vi "comDBPatientQueries.vi"(0 "id":string, 1 "State":T1, 2 "select":enum16{"Default", "Trash", "Training"}(ring), 5 "입력":string[](array[string]), 7 "searchForm":string, 9 "crrentPage":string, 11 "error in (no error)":errorcluster caption="에러 입력(에러 없음)") -> (4 "resultList":string[][](table) caption="result2DArray", 6 "result1DArray":string[](array[string]), 8 "count":i64, 15 "error out":errorcluster caption="에러 출력")   [LabVIEW 2019]
uses:
  patients_state.ctl
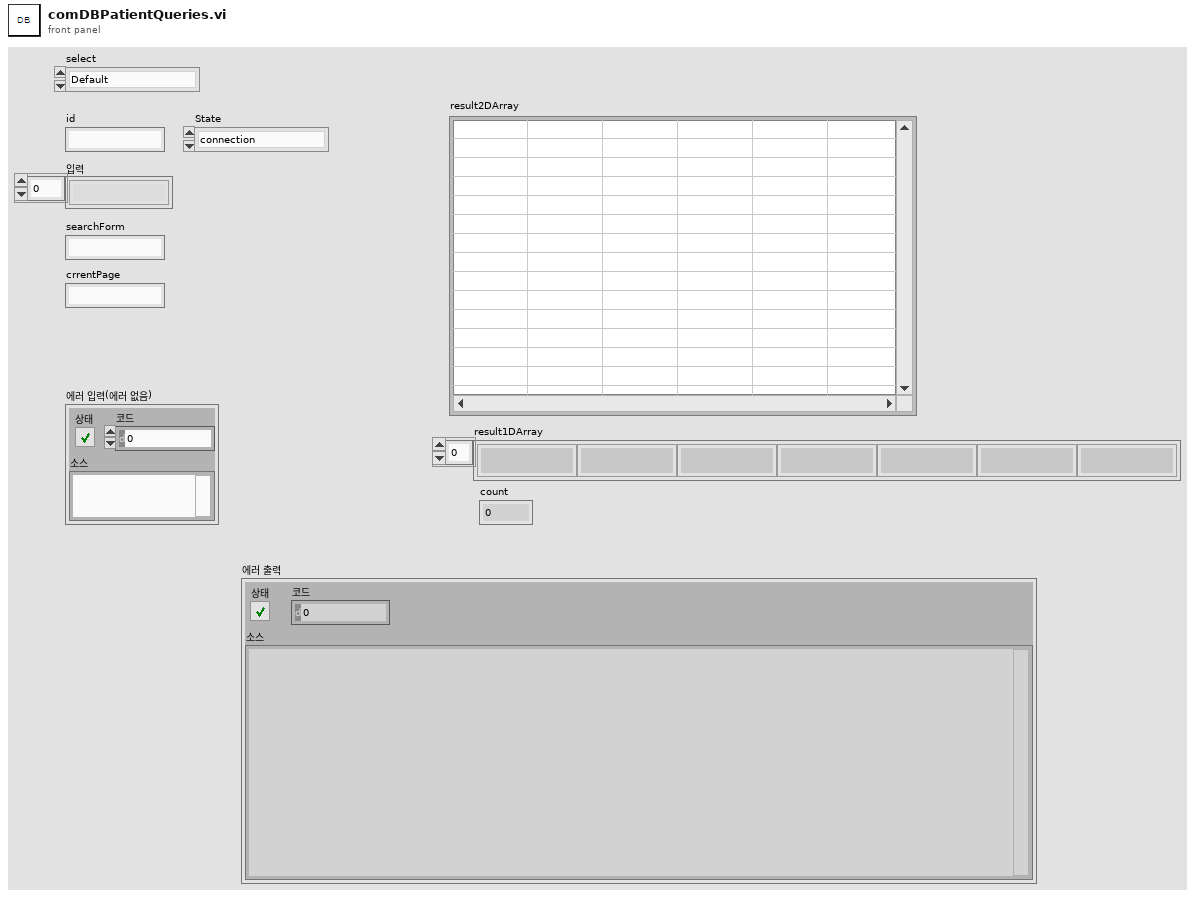
[diagram p1: front panel]
types:
  T1 = typedef "patients_state.ctl" = enum16{"connection", "create", "getReadList", "getRead", "getCount", "update", "delete", "trash", "restore", "close"}
  T2 = enum16{"connection", "create", "getReadList", "getRead", "getCount", "update", "delete", "close"}
  T3 = enum16{"connection", "create", "read", "update", "delete", "close"}
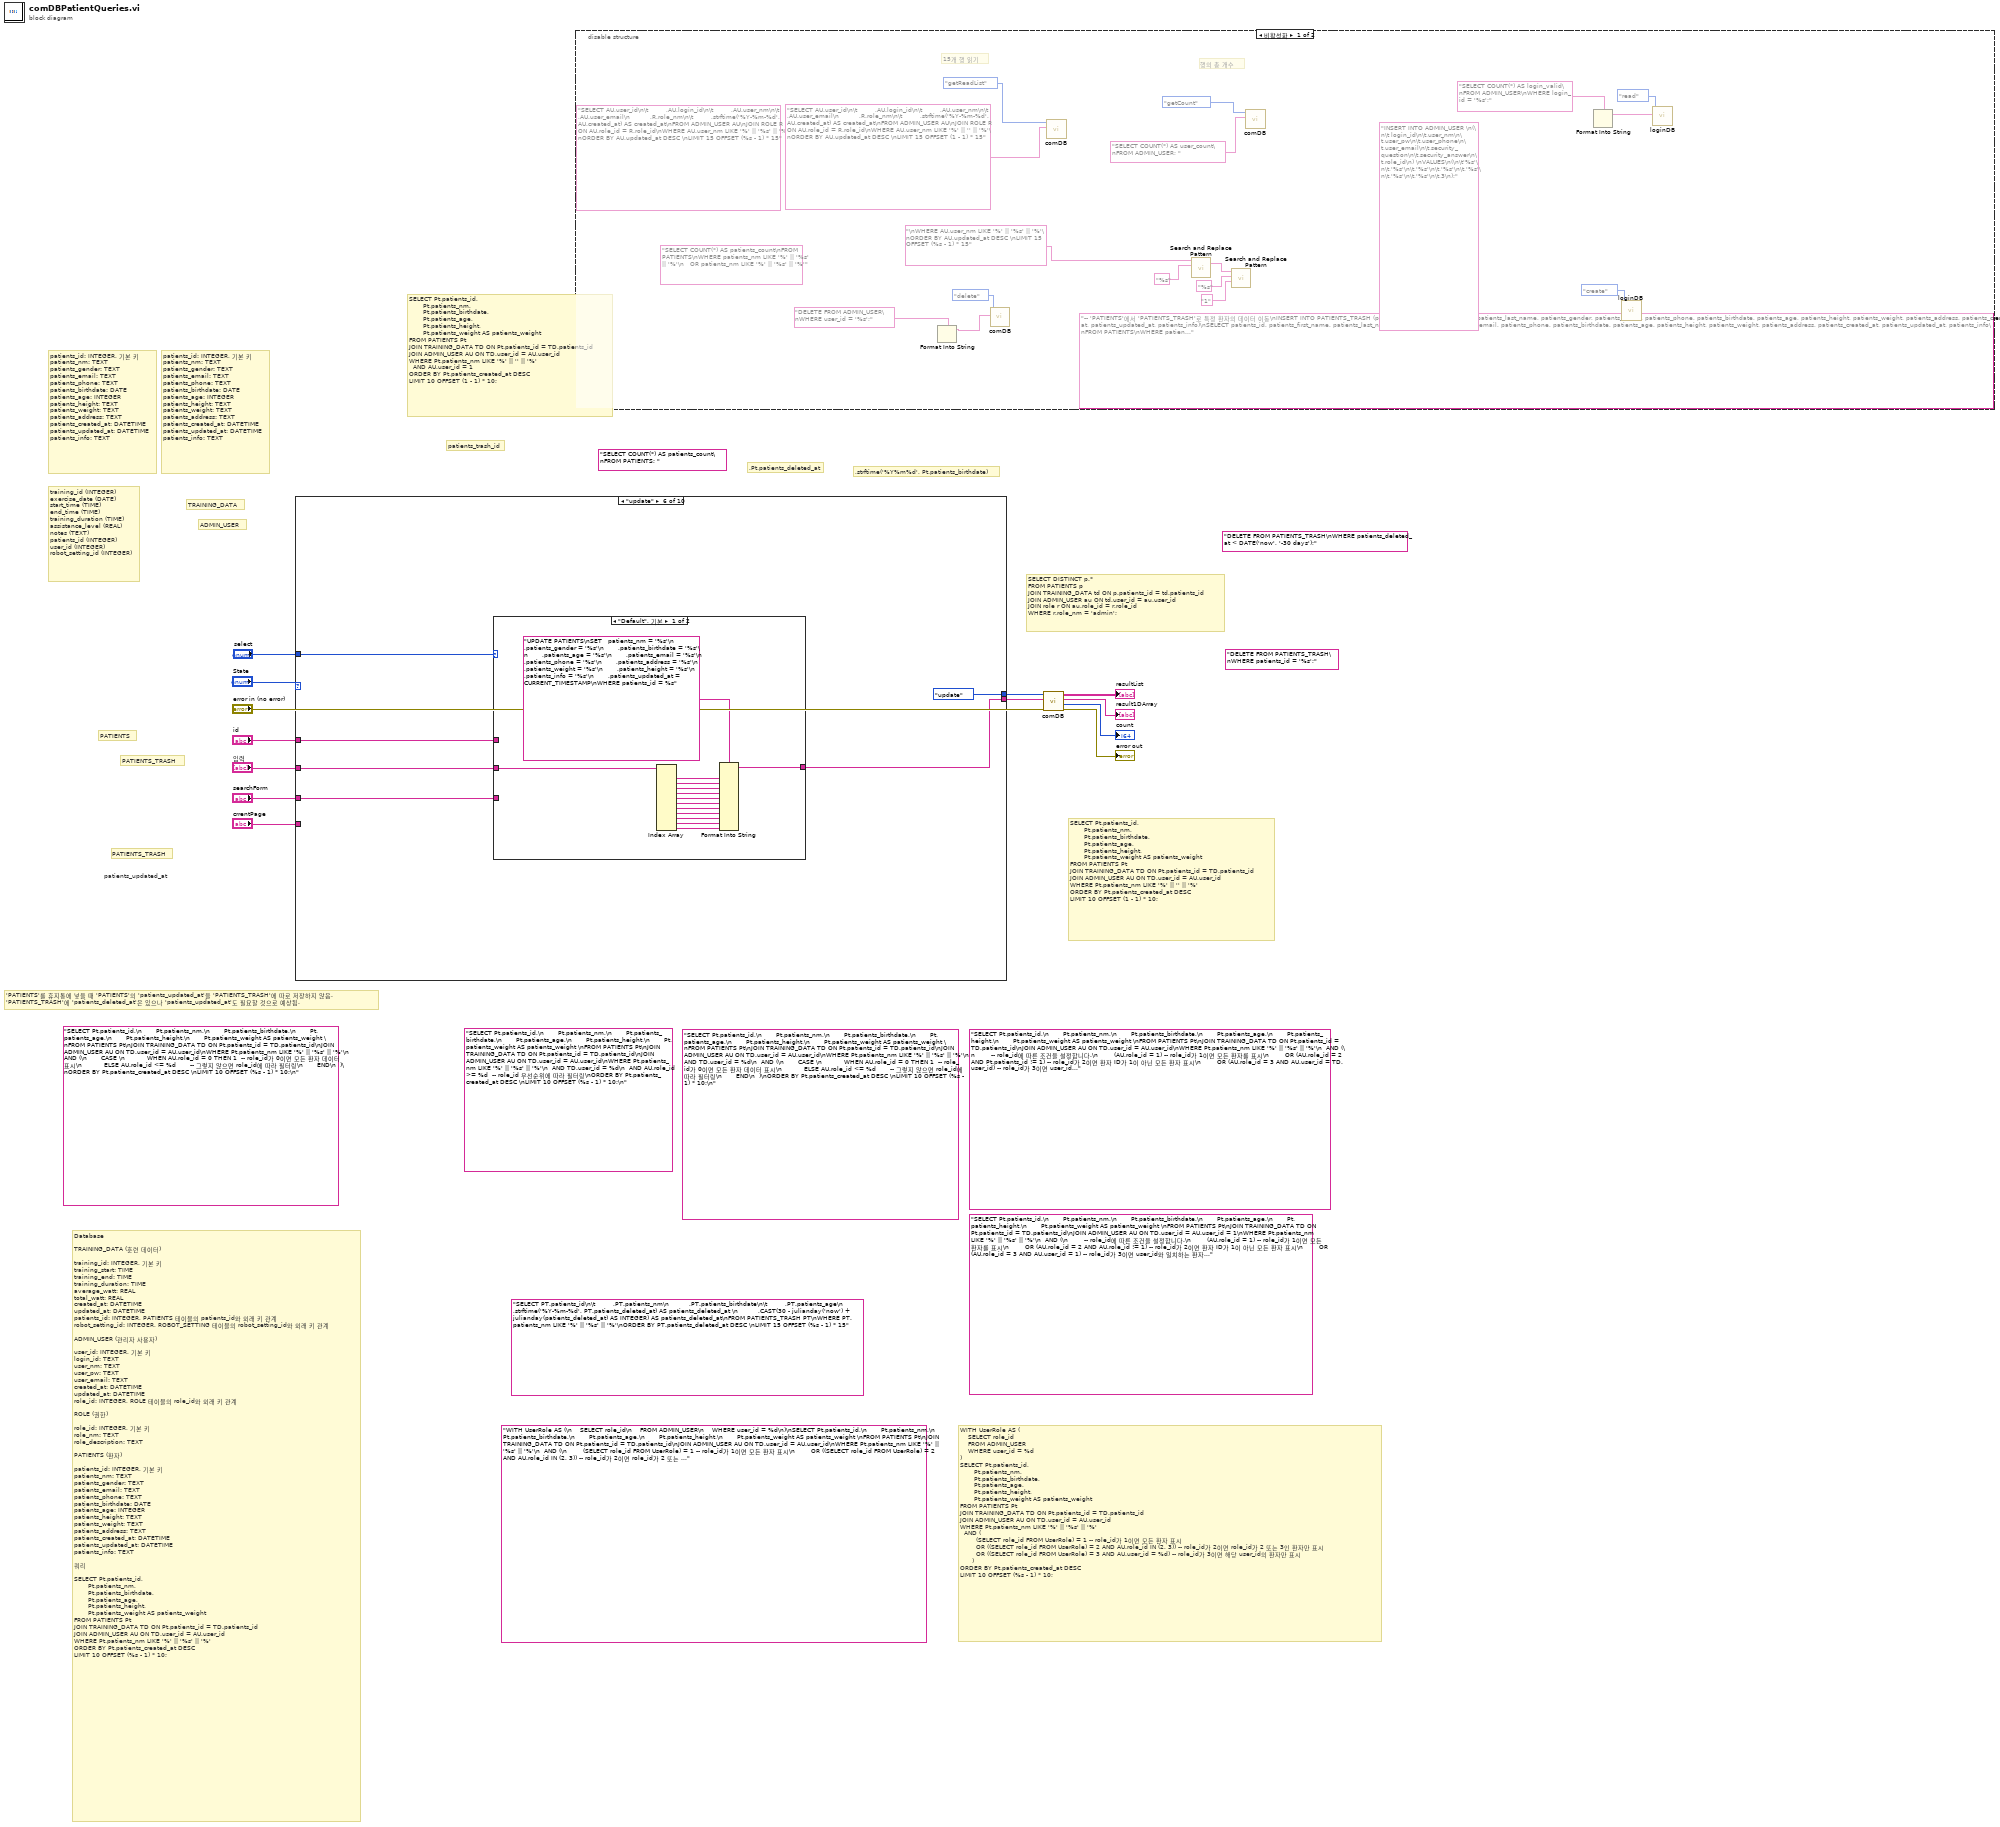
[diagram p0: block diagram]
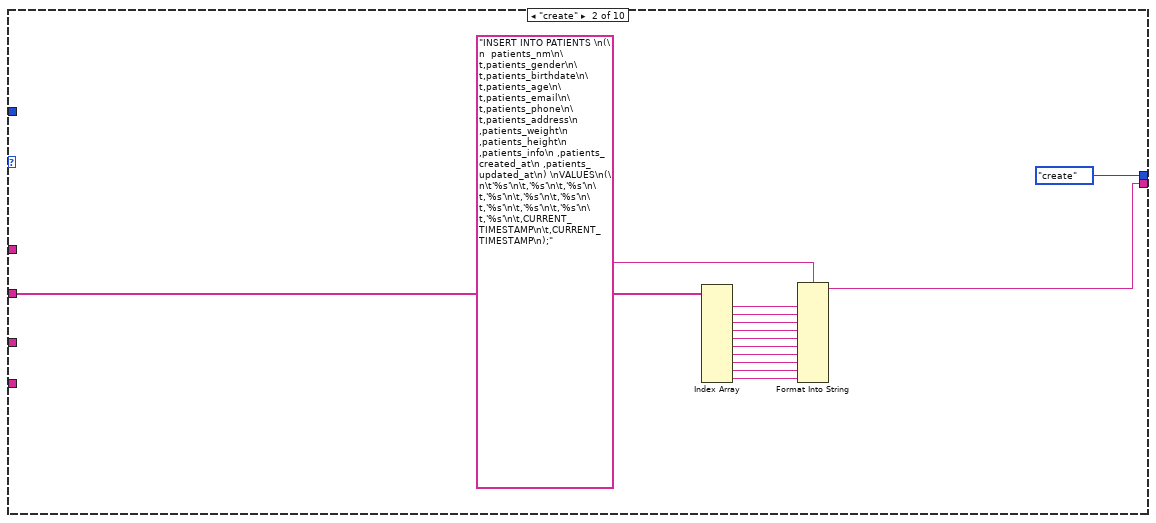
[diagram p3: hidden frame]
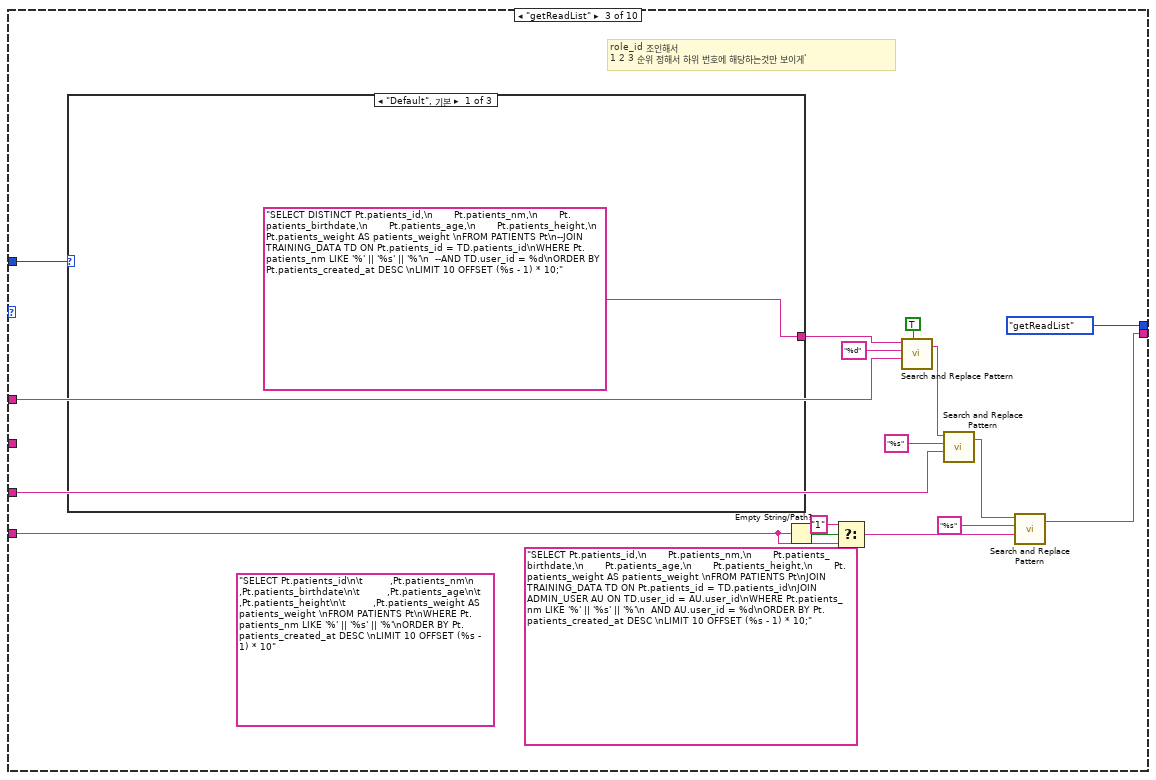
[diagram p4: hidden frame]
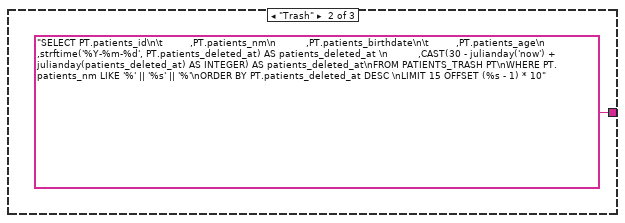
[diagram p5: hidden frame]
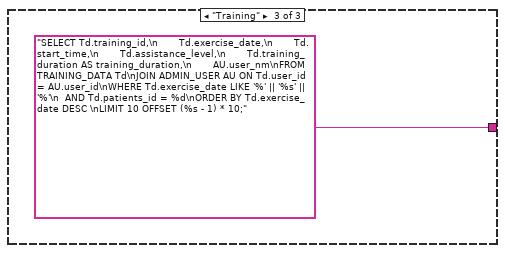
[diagram p6: hidden frame]
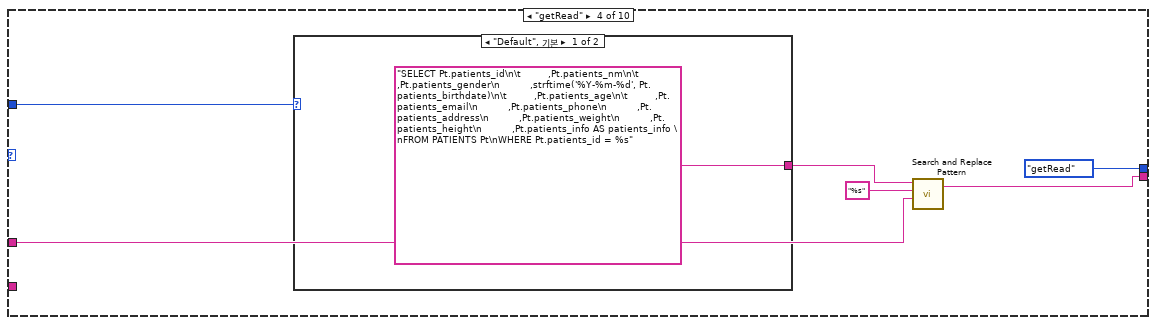
[diagram p7: hidden frame]
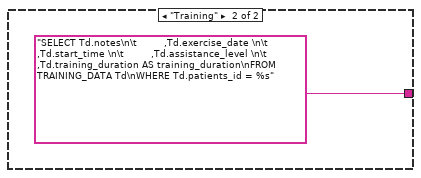
[diagram p8: hidden frame]
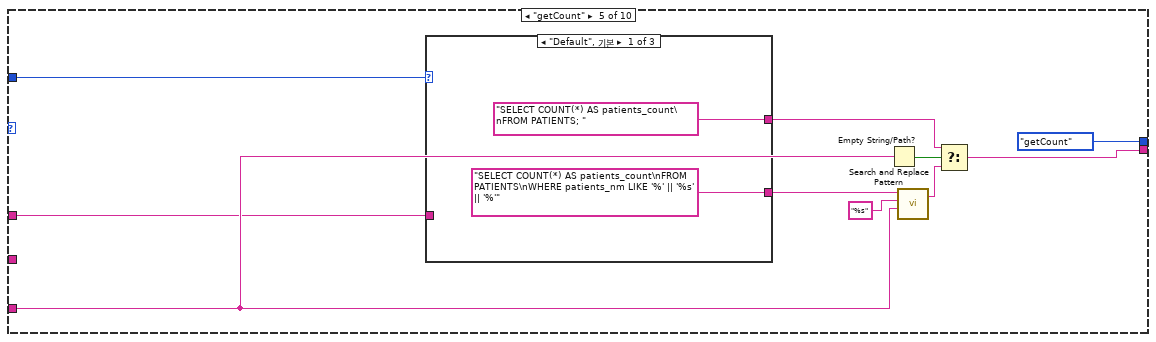
[diagram p9: hidden frame]
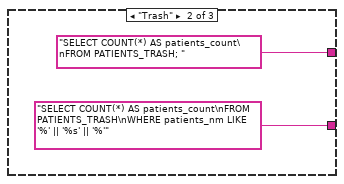
[diagram p10: hidden frame]
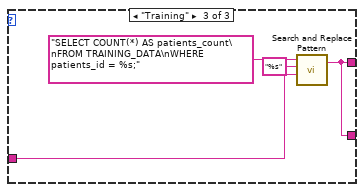
[diagram p11: hidden frame]
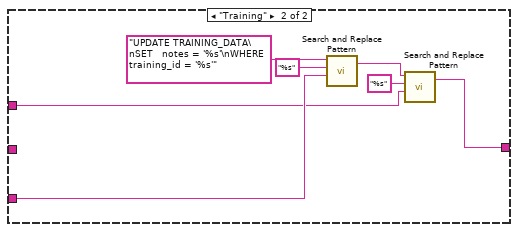
[diagram p12: hidden frame]
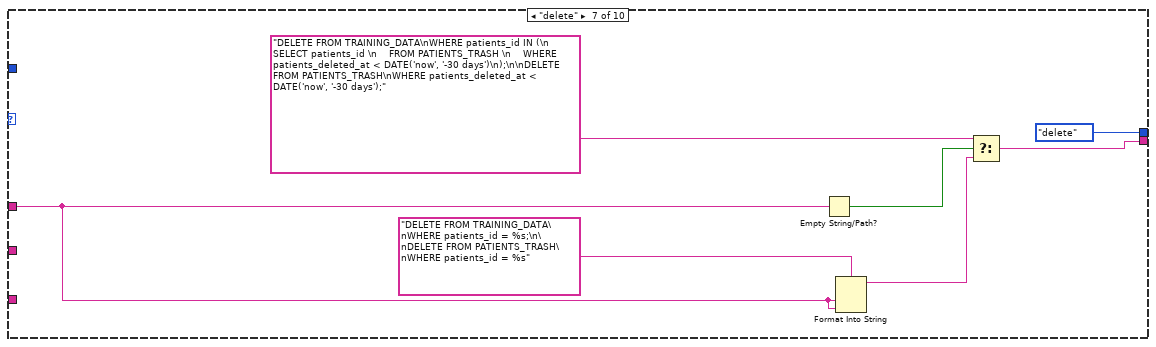
[diagram p13: hidden frame]
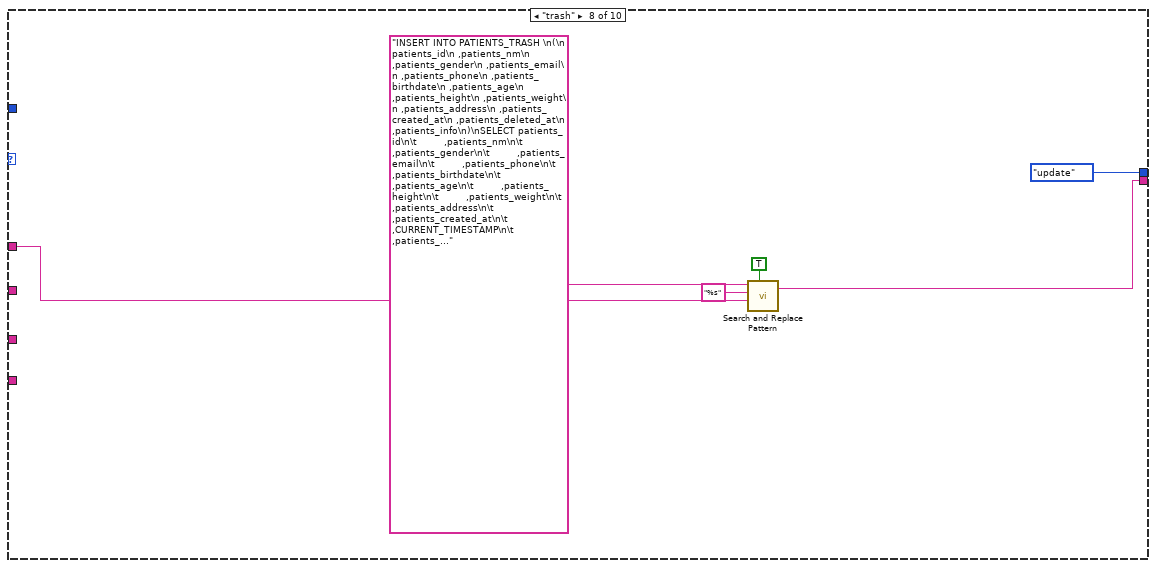
[diagram p14: hidden frame]
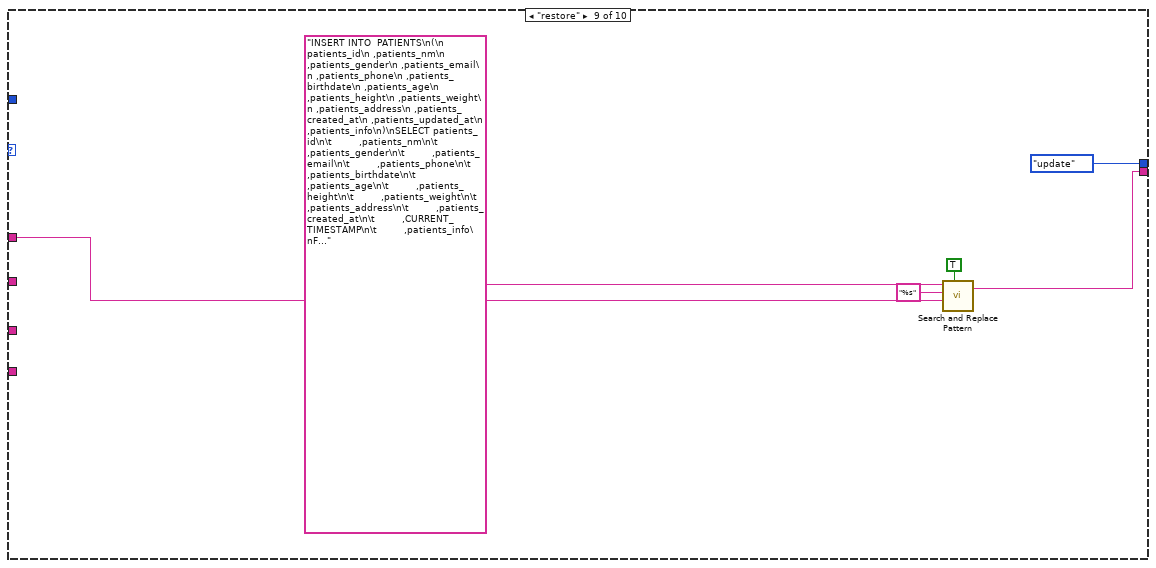
[diagram p15: hidden frame]
diagram:
  (unwired) "WITH UserRole AS (\n    SELECT role_id\n    FROM ADMIN_USER\n    WHERE user_id = %d\n)\nSELECT Pt.patients_id,\n       Pt.patients_nm,\n       Pt.patients_birthdate,\n       Pt.patients_age,\n       Pt.patients_height,\n       Pt.patients_weight AS patients_weight \nFROM PATIENTS Pt\nJOIN TRAINING_DATA TD ON Pt.patients_id = TD.patients_id\nJOIN ADMIN_USER AU ON TD.user_id = AU.user_id\nWHERE Pt.patients_nm LIKE '%' || '%s' || '%'\n  AND (\n        (SELECT role_id FROM UserRole) = 1 -- role_id가 1이면 모든 환자 표시\n        OR ((SELECT role_id FROM UserRole) = 2 AND AU.role_id IN (2, 3)) -- role_id가 2이면 role_id가 2 또는 3인 환자만 표시\n        OR ((SELECT role_id FROM UserRole) = 3 AND AU.user_id = %d) -- role_id가 3이면 해당 user_id의 환자만 표시\n      )\nORDER BY Pt.patients_created_at DESC \nLIMIT 10 OFFSET (%s - 1) * 10;\n" ("Query")
  (unwired) "SELECT PT.patients_id\n\t         ,PT.patients_nm\n          ,PT.patients_birthdate\n\t         ,PT.patients_age\n          ,strftime('%Y-%m-%d', PT.patients_deleted_at) AS patients_deleted_at \n          ,CAST(30 - julianday('now') + julianday(patients_deleted_at) AS INTEGER) AS patients_deleted_at\nFROM PATIENTS_TRASH PT\nWHERE PT.patients_nm LIKE '%' || '%s' || '%'\nORDER BY PT.patients_deleted_at DESC \nLIMIT 15 OFFSET (%s - 1) * 15" ("Query")
  (unwired) "SELECT Pt.patients_id,\n       Pt.patients_nm,\n       Pt.patients_birthdate,\n       Pt.patients_age,\n       Pt.patients_height,\n       Pt.patients_weight AS patients_weight \nFROM PATIENTS Pt\nJOIN TRAINING_DATA TD ON Pt.patients_id = TD.patients_id\nJOIN ADMIN_USER AU ON TD.user_id = AU.user_id = 1\nWHERE Pt.patients_nm LIKE '%' || '%s' || '%'\n  AND (\n        -- role_id에 따른 조건을 설정합니다.\n        (AU.role_id = 1) -- role_id가 1이면 모든 환자를 표시\n        OR (AU.role_id = 2 AND AU.role_id != 1) -- role_id가 2이면 환자 ID가 1이 아닌 모든 환자 표시\n        OR (AU.role_id = 3 AND AU.user_id = 1) -- role_id가 3이면 user_id와 일치하는 환자만 표시\n      )\nORDER BY Pt.patients_created_at DESC \nLIMIT 10 OFFSET (%s - 1) * 10;\n" ("Query")
  (unwired) "SELECT Pt.patients_id,\n       Pt.patients_nm,\n       Pt.patients_birthdate,\n       Pt.patients_age,\n       Pt.patients_height,\n       Pt.patients_weight AS patients_weight \nFROM PATIENTS Pt\nJOIN TRAINING_DATA TD ON Pt.patients_id = TD.patients_id\nJOIN ADMIN_USER AU ON TD.user_id = AU.user_id\nWHERE Pt.patients_nm LIKE '%' || '%s' || '%'\n  AND (\n        -- role_id에 따른 조건을 설정합니다.\n        (AU.role_id = 1) -- role_id가 1이면 모든 환자를 표시\n        OR (AU.role_id = 2 AND Pt.patients_id != 1) -- role_id가 2이면 환자 ID가 1이 아닌 모든 환자 표시\n        OR (AU.role_id = 3 AND AU.user_id = TD.user_id) -- role_id가 3이면 user_id와 일치하는 환자만 표시\n      )\nORDER BY Pt.patients_created_at DESC \nLIMIT 10 OFFSET (%s - 1) * 10;\n" ("Query")
  (unwired) "SELECT Pt.patients_id,\n       Pt.patients_nm,\n       Pt.patients_birthdate,\n       Pt.patients_age,\n       Pt.patients_height,\n       Pt.patients_weight AS patients_weight \nFROM PATIENTS Pt\nJOIN TRAINING_DATA TD ON Pt.patients_id = TD.patients_id\nJOIN ADMIN_USER AU ON TD.user_id = AU.user_id\nWHERE Pt.patients_nm LIKE '%' || '%s' || '%'\n  AND (\n       CASE \n           WHEN AU.role_id = 0 THEN 1  -- role_id가 0이면 모든 환자 데이터 표시\n           ELSE AU.role_id <= %d       -- 그렇지 않으면 role_id에 따라 필터링\n       END\n  )\nORDER BY Pt.patients_created_at DESC \nLIMIT 10 OFFSET (%s - 1) * 10;\n" ("Query")
  (unwired) "SELECT Pt.patients_id,\n       Pt.patients_nm,\n       Pt.patients_birthdate,\n       Pt.patients_age,\n       Pt.patients_height,\n       Pt.patients_weight AS patients_weight \nFROM PATIENTS Pt\nJOIN TRAINING_DATA TD ON Pt.patients_id = TD.patients_id\nJOIN ADMIN_USER AU ON TD.user_id = AU.user_id\nWHERE Pt.patients_nm LIKE '%' || '%s' || '%'\n  AND TD.user_id = %d\n  AND (\n       CASE \n           WHEN AU.role_id = 0 THEN 1  -- role_id가 0이면 모든 환자 데이터 표시\n           ELSE AU.role_id <= %d       -- 그렇지 않으면 role_id에 따라 필터링\n       END\n  )\nORDER BY Pt.patients_created_at DESC \nLIMIT 10 OFFSET (%s - 1) * 10;\n" ("Query")
  (unwired) "SELECT Pt.patients_id,\n       Pt.patients_nm,\n       Pt.patients_birthdate,\n       Pt.patients_age,\n       Pt.patients_height,\n       Pt.patients_weight AS patients_weight \nFROM PATIENTS Pt\nJOIN TRAINING_DATA TD ON Pt.patients_id = TD.patients_id\nJOIN ADMIN_USER AU ON TD.user_id = AU.user_id\nWHERE Pt.patients_nm LIKE '%' || '%s' || '%'\n  AND TD.user_id = %d\n  AND AU.role_id >= %d  -- role_id 우선순위에 따라 필터링\nORDER BY Pt.patients_created_at DESC \nLIMIT 10 OFFSET (%s - 1) * 10;\n" ("Query")
  (unwired) "DELETE FROM PATIENTS_TRASH\nWHERE patients_id = '%s';" ("Query")
  (unwired) "DELETE FROM PATIENTS_TRASH\nWHERE patients_deleted_at < DATE('now', '-30 days');" ("Query")
  (unwired) "SELECT COUNT(*) AS patients_count\nFROM PATIENTS; " ("Query")
  # "SELECT DISTINCT p.*\nFROM PATIENTS p\nJOIN TRAINING_DATA td ON p.patients_id = td.patients_id\nJOIN ADMIN_USER au ON td.user_id = au.user_id\nJOIN role r ON au.role_id = r.role_id\nWHERE r.role_nm = 'admin';"
  # "X"
  # "X"
  # "X"
  # "X"
  # "X"
  # "X"
  # "SELECT Pt.patients_id,\n       Pt.patients_nm,\n       Pt.patients_birthdate,\n       Pt.patients_age,\n       Pt.patients_height,\n       Pt.patients_weight AS patients_weight \nFROM PATIENTS Pt\nJOIN TRAINING_DATA TD ON Pt.patients_id = TD.patients_id\nJOIN ADMIN_USER AU ON TD.user_id = AU.user_id\nWHERE Pt.patients_nm LIKE '%' || '' || '%'\nORDER BY Pt.patients_created_at DESC \nLIMIT 10 OFFSET (1 - 1) * 10;"
  # "WITH UserRole AS (\n    SELECT role_id\n    FROM ADMIN_USER\n    WHERE user_id = %d\n)\nSELECT Pt.patients_id,\n       Pt.patients_nm,\n       Pt.patients_birthdate,\n       Pt.patients_age,\n       Pt.patients_height,\n       Pt.patients_weight AS patients_weight \nFROM PATIENTS Pt\nJOIN TRAINING_DATA TD ON Pt.patients_id = TD.patients_id\nJOIN ADMIN_USER AU ON TD.user_id = AU.user_id\nWHERE Pt.patients_nm LIKE '%' || '%s' || '%'\n  AND (\n        (SELECT role_id FROM UserRole) = 1 -- role_id가 1이면 모든 환자 표시\n        OR ((SELECT role_id FROM UserRole) = 2 AND AU.role_id IN (2, 3)) -- role_id가 2이면 role_id가 2 또는 3인 환자만 표시\n        OR ((SELECT role_id FROM UserRole) = 3 AND AU.user_id = %d) -- role_id가 3이면 해당 user_id의 환자만 표시\n      )\nORDER BY Pt.patients_created_at DESC \nLIMIT 10 OFFSET (%s - 1) * 10;"
  # "Database\n\nTRAINING_DATA (훈련 데이터)\n\ntraining_id: INTEGER, 기본 키\ntraining_start: TIME\ntraining_end: TIME\ntraining_duration: TIME\naverage_watt: REAL\ntotal_watt: REAL\ncreated_at: DATETIME\nupdated_at: DATETIME\npatients_id: INTEGER, PATIENTS 테이블의 patients_id와 외래 키 관계\nrobot_setting_id: INTEGER, ROBOT_SETTING 테이블의 robot_setting_id와 외래 키 관계\n\nADMIN_USER (관리자 사용자)\n\nuser_id: INTEGER, 기본 키\nlogin_id: TEXT\nuser_nm: TEXT\nuser_pw: TEXT\nuser_email: TEXT\ncreated_at: DATETIME\nupdated_at: DATETIME\nrole_id: INTEGER, ROLE 테이블의 role_id와 외래 키 관계\n\nROLE (권한)\n\nrole_id: INTEGER, 기본 키\nrole_nm: TEXT\nrole_description: TEXT\n\nPATIENTS (환자)\n\npatients_id: INTEGER, 기본 키\npatients_nm: TEXT\npatients_gender: TEXT\npatients_email: TEXT\npatients_phone: TEXT\npatients_birthdate: DATE\npatients_age: INTEGER\npatients_height: TEXT\npatients_weight: TEXT\npatients_address: TEXT\npatients_created_at: DATETIME\npatients_updated_at: DATETIME\npatients_info: TEXT\n\n쿼리\n\nSELECT Pt.patients_id,\n       Pt.patients_nm,\n       Pt.patients_birthdate,\n       Pt.patients_age,\n       Pt.patients_height,\n       Pt.patients_weight AS patients_weight \nFROM PATIENTS Pt\nJOIN TRAINING_DATA TD ON Pt.patients_id = TD.patients_id\nJOIN ADMIN_USER AU ON TD.user_id = AU.user_id\nWHERE Pt.patients_nm LIKE '%' || '%s' || '%'\nORDER BY Pt.patients_created_at DESC \nLIMIT 10 OFFSET (%s - 1) * 10;"
  # "SELECT Pt.patients_id,\n       Pt.patients_nm,\n       Pt.patients_birthdate,\n       Pt.patients_age,\n       Pt.patients_height,\n       Pt.patients_weight AS patients_weight \nFROM PATIENTS Pt\nJOIN TRAINING_DATA TD ON Pt.patients_id = TD.patients_id\nJOIN ADMIN_USER AU ON TD.user_id = AU.user_id\nWHERE Pt.patients_nm LIKE '%' || '' || '%'\n  AND AU.user_id = 1\nORDER BY Pt.patients_created_at DESC \nLIMIT 10 OFFSET (1 - 1) * 10;"
  # "ADMIN_USER"
  # "patients_trash_id"
  # "TRAINING_DATA"
  # "training_id (INTEGER)\nexercise_date (DATE)\nstart_time (TIME)\nend_time (TIME)\ntraining_duration (TIME)\nassistance_level (REAL)\nnotes (TEXT)\npatients_id (INTEGER)\nuser_id (INTEGER)\nrobot_setting_id (INTEGER)"
  # ",Pt.patients_deleted_at"
  # ",strftime('%Y%m%d', Pt.patients_birthdate)"
  # "patients_updated_at"
  # "PATIENTS_TRASH"
  # "'PATIENTS'를 휴지통에 넣을 때 'PATIENTS'의 'patients_updated_at'을 'PATIENTS_TRASH'에 따로 저장하지 않음.\n'PATIENTS_TRASH'에 'patients_deleted_at'은 있으나 'patients_updated_at'도 필요할 것으로 예상됨."
  # "patients_id: INTEGER, 기본 키\npatients_nm: TEXT\npatients_gender: TEXT\npatients_email: TEXT\npatients_phone: TEXT\npatients_birthdate: DATE\npatients_age: INTEGER\npatients_height: TEXT\npatients_weight: TEXT\npatients_address: TEXT\npatients_created_at: DATETIME\npatients_updated_at: DATETIME\npatients_info: TEXT"
  # "PATIENTS_TRASH"
  # "PATIENTS"
  # "patients_id: INTEGER, 기본 키\npatients_nm: TEXT\npatients_gender: TEXT\npatients_email: TEXT\npatients_phone: TEXT\npatients_birthdate: DATE\npatients_age: INTEGER\npatients_height: TEXT\npatients_weight: TEXT\npatients_address: TEXT\npatients_created_at: DATETIME\npatients_updated_at: DATETIME\npatients_info: TEXT"
  n1 = case shown="\"update\"" "State" {
    tunnel: [_ T2."create" ("State") T2."getReadList" ("State") T2."getRead" ("State") T2."getCount" ("State") T2."update" ("State") T2."delete" ("State") T2."update" ("State") T2."update" ("State") _] -> w11
    tunnel: [_ w17 w38 w49 w60 w76 w102 w109 w114 _] -> w10
    tunnel: "searchForm" -> [_ _ w41 _ w59 w73 _ _ _ _]
    tunnel: "crrentPage" -> [_ _ w35 _ _ _ _ _ _ _]
    tunnel: "id" -> [_ _ w30 w50 w55 w74 w100 w107 w115 _]
    tunnel: "입력" -> [_ w19 _ _ _ w77 _ _ _ _]
    tunnel: "select" -> [_ _ w33 w48 w58 w75 _ _ _ _]
    frame "connection", Default {
      # "x"
    }
    frame "create" {
      n2 = Index Array(array=w19) -> (element #1=w26:string, element #2=w25:string, element #3=w24:string, element #4=w23:string, element #5=w22:string, element #6=w21:string, element #7=w20:string, element #8=w16:string, element #9=w15:string, element #10=w14:string)  [unwired: 10 in]
      n3 = Format Into String(format string="INSERT INTO PATIENTS \n(\n  patients_nm\n\t,patients_gender\n\t,patients_birthdate\n\t,patients_age\n\t,patients_email\n\t,patients_phone\n\t,patients_address\n ,patients_weight\n ,patients_height\n ,patients_info\n ,patients_created_at\n ,patients_updated_at\n) \nVALUES\n(\n\t'%s'\n\t,'%s'\n\t,'%s'\n\t,'%s'\n\t,'%s'\n\t,'%s'\n\t,'%s'\n\t,'%s'\n\t,'%s'\n\t,'%s'\n\t,CURRENT_TIMESTAMP\n\t,CURRENT_TIMESTAMP\n);", w26, w25, w24, w23, w22, w21, w20, w16, w15, w14) -> (resulting string=w17:string)  [unwired: 2 in, 1 out]
    }
    frame "getReadList" {
      (unwired) "SELECT Pt.patients_id,\n       Pt.patients_nm,\n       Pt.patients_birthdate,\n       Pt.patients_age,\n       Pt.patients_height,\n       Pt.patients_weight AS patients_weight \nFROM PATIENTS Pt\nJOIN TRAINING_DATA TD ON Pt.patients_id = TD.patients_id\nJOIN ADMIN_USER AU ON TD.user_id = AU.user_id\nWHERE Pt.patients_nm LIKE '%' || '%s' || '%'\n  AND AU.user_id = %d\nORDER BY Pt.patients_created_at DESC \nLIMIT 10 OFFSET (%s - 1) * 10;" ("Query")
      (unwired) "SELECT Pt.patients_id\n\t         ,Pt.patients_nm\n          ,Pt.patients_birthdate\n\t         ,Pt.patients_age\n\t         ,Pt.patients_height\n\t         ,Pt.patients_weight AS patients_weight \nFROM PATIENTS Pt\nWHERE Pt.patients_nm LIKE '%' || '%s' || '%'\nORDER BY Pt.patients_created_at DESC \nLIMIT 10 OFFSET (%s - 1) * 10" ("Query")
      # "role_id 조인해서 \n1 2 3 순위 정해서 하위 번호에 해당하는것만 보이게'"
      n4 = case shown="\"Default\", 기본" w33 {
        tunnel: ["SELECT DISTINCT Pt.patients_id,\n       Pt.patients_nm,\n       Pt.patients_birthdate,\n       Pt.patients_age,\n       Pt.patients_height,\n       Pt.patients_weight AS patients_weight \nFROM PATIENTS Pt\n--JOIN TRAINING_DATA TD ON Pt.patients_id = TD.patients_id\nWHERE Pt.patients_nm LIKE '%' || '%s' || '%'\n  --AND TD.user_id = %d\nORDER BY Pt.patients_created_at DESC \nLIMIT 10 OFFSET (%s - 1) * 10;" ("Query") "SELECT PT.patients_id\n\t         ,PT.patients_nm\n          ,PT.patients_birthdate\n\t         ,PT.patients_age\n          ,strftime('%Y-%m-%d', PT.patients_deleted_at) AS patients_deleted_at \n          ,CAST(30 - julianday('now') + julianday(patients_deleted_at) AS INTEGER) AS patients_deleted_at\nFROM PATIENTS_TRASH PT\nWHERE PT.patients_nm LIKE '%' || '%s' || '%'\nORDER BY PT.patients_deleted_at DESC \nLIMIT 15 OFFSET (%s - 1) * 10" ("Query") "SELECT Td.training_id,\n       Td.exercise_date,\n       Td.start_time,\n       Td.assistance_level,\n       Td.training_duration AS training_duration,\n       AU.user_nm\nFROM TRAINING_DATA Td\nJOIN ADMIN_USER AU ON Td.user_id = AU.user_id\nWHERE Td.exercise_date LIKE '%' || '%s' || '%'\n  AND Td.patients_id = %d\nORDER BY Td.exercise_date DESC \nLIMIT 10 OFFSET (%s - 1) * 10;" ("Query")] -> w32
        frame "Default", Default {
        }
        frame "Trash" {
        }
        frame "Training" {
        }
      }
      n5 = Empty String/Path?(string/path=w35) -> (empty?=w37:bool)
      n6 = Select(t="1", s=w37, f=w35) -> (s? t:f=w36:string)
      n7 = call <vilib>:"Search and Replace Pattern.vi"("string"=w32, "regular expression (\"\")"="%d" ("regular expression (\"\")"), "replace string (\"\")"=w30, "replace all? (F)"=TRUE) -> ("result string"=w29:string)  [unwired: 1 in, 1 out]
      n8 = call <vilib>:"Search and Replace Pattern.vi"("string"=w29, "regular expression (\"\")"="%s" ("regular expression (\"\")"), "replace string (\"\")"=w41) -> ("result string"=w39:string)  [unwired: 2 in, 1 out]
      n9 = call <vilib>:"Search and Replace Pattern.vi"("string"=w39, "regular expression (\"\")"="%s" ("regular expression (\"\")"), "replace string (\"\")"=w36) -> ("result string"=w38:string)  [unwired: 2 in, 1 out]
    }
    frame "getRead" {
      n10 = case shown="\"Default\", 기본" w48 {
        tunnel: ["SELECT Pt.patients_id\n\t         ,Pt.patients_nm\n\t         ,Pt.patients_gender\n          ,strftime('%Y-%m-%d', Pt.patients_birthdate)\n\t         ,Pt.patients_age\n\t         ,Pt.patients_email\n          ,Pt.patients_phone\n          ,Pt.patients_address\n          ,Pt.patients_weight\n          ,Pt.patients_height\n          ,Pt.patients_info AS patients_info \nFROM PATIENTS Pt\nWHERE Pt.patients_id = %s" ("Query") "SELECT Td.notes\n\t         ,Td.exercise_date \n\t         ,Td.start_time \n\t         ,Td.assistance_level \n\t         ,Td.training_duration AS training_duration\nFROM TRAINING_DATA Td\nWHERE Td.patients_id = %s" ("Query")] -> w47
        frame "Default", Default {
        }
        frame "Training" {
        }
      }
      n11 = call <vilib>:"Search and Replace Pattern.vi"("string"=w47, "regular expression (\"\")"="%s" ("regular expression (\"\")"), "replace string (\"\")"=w50) -> ("result string"=w49:string)  [unwired: 2 in, 1 out]
    }
    frame "getCount" {
      n12 = case shown="\"Default\", 기본" w58 {
        tunnel: ["SELECT COUNT(*) AS patients_count\nFROM PATIENTS; " ("Query") "SELECT COUNT(*) AS patients_count\nFROM PATIENTS_TRASH; " ("Query") w69] -> w57
        tunnel: ["SELECT COUNT(*) AS patients_count\nFROM PATIENTS\nWHERE patients_nm LIKE '%' || '%s' || '%'" ("Query") "SELECT COUNT(*) AS patients_count\nFROM PATIENTS_TRASH\nWHERE patients_nm LIKE '%' || '%s' || '%'" ("Query") w69] -> w56
        tunnel: w55 -> [_ _ w70]
        frame "Default", Default {
        }
        frame "Trash" {
        }
        frame "Training" {
          n13 = call <vilib>:"Search and Replace Pattern.vi"("string"="SELECT COUNT(*) AS patients_count\nFROM TRAINING_DATA\nWHERE patients_id = %s;" ("Query"), "regular expression (\"\")"="%s" ("regular expression (\"\")"), "replace string (\"\")"=w70) -> ("result string"=w69:string)  [unwired: 2 in, 1 out]
        }
      }
      n14 = Empty String/Path?(string/path=w59) -> (empty?=w63:bool)
      n15 = call <vilib>:"Search and Replace Pattern.vi"("string"=w56, "regular expression (\"\")"="%s" ("regular expression (\"\")"), "replace string (\"\")"=w59) -> ("result string"=w61:string)  [unwired: 2 in, 1 out]
      n16 = Select(t=w57, s=w63, f=w61) -> (s? t:f=w60:string)
    }
    frame "update" {
      n17 = case shown="\"Default\", 기본" w75 {
        tunnel: w77 -> [w92 _]
        tunnel: [w83 w93] -> w76
        tunnel: w74 -> [_ w94]
        tunnel: w73 -> [_ w96]
        frame "Default", Default {
          n18 = Index Array(array=w92) -> (element #1=w91:string, element #2=w90:string, element #3=w89:string, element #4=w88:string, element #5=w87:string, element #6=w86:string, element #7=w85:string, element #8=w82:string, element #9=w81:string, element #10=w80:string, element #11=w79:string)  [unwired: 11 in]
          n19 = Format Into String(format string="UPDATE PATIENTS\nSET   patients_nm = '%s'\n       ,patients_gender = '%s'\n       ,patients_birthdate = '%s'\n       ,patients_age = '%s'\n       ,patients_email = '%s'\n       ,patients_phone = '%s'\n       ,patients_address = '%s'\n       ,patients_weight = '%s'\n       ,patients_height = '%s'\n       ,patients_info = '%s'\n       ,patients_updated_at = CURRENT_TIMESTAMP\nWHERE patients_id = %s" ("Query"), w91, w90, w89, w88, w87, w86, w85, w82, w81, w80, w79) -> (resulting string=w83:string)  [unwired: 2 in, 1 out]
        }
        frame "Training" {
          n20 = call <vilib>:"Search and Replace Pattern.vi"("string"="UPDATE TRAINING_DATA\nSET   notes = '%s'\nWHERE training_id = '%s'" ("Query"), "regular expression (\"\")"="%s" ("regular expression (\"\")"), "replace string (\"\")"=w96) -> ("result string"=w95:string)  [unwired: 2 in, 1 out]
          n21 = call <vilib>:"Search and Replace Pattern.vi"("string"=w95, "regular expression (\"\")"="%s" ("regular expression (\"\")"), "replace string (\"\")"=w94) -> ("result string"=w93:string)  [unwired: 2 in, 1 out]
        }
      }
    }
    frame "delete" {
      n22 = Empty String/Path?(string/path=w100) -> (empty?=w104:bool)
      n23 = Format Into String(format string="DELETE FROM TRAINING_DATA\nWHERE patients_id = %s;\n\nDELETE FROM PATIENTS_TRASH\nWHERE patients_id = %s" ("Query"), w100, w100) -> (resulting string=w103:string)  [unwired: 2 in, 1 out]
      n24 = Select(t="DELETE FROM TRAINING_DATA\nWHERE patients_id IN (\n    SELECT patients_id \n    FROM PATIENTS_TRASH \n    WHERE patients_deleted_at < DATE('now', '-30 days')\n);\n\nDELETE FROM PATIENTS_TRASH\nWHERE patients_deleted_at < DATE('now', '-30 days');" ("Query"), s=w104, f=w103) -> (s? t:f=w102:string)
    }
    frame "trash" {
      n25 = call <vilib>:"Search and Replace Pattern.vi"("string"="INSERT INTO PATIENTS_TRASH \n(\n  patients_id\n ,patients_nm\n ,patients_gender\n ,patients_email\n ,patients_phone\n ,patients_birthdate\n ,patients_age\n ,patients_height\n ,patients_weight\n ,patients_address\n ,patients_created_at\n ,patients_deleted_at\n ,patients_info\n)\nSELECT patients_id\n\t         ,patients_nm\n\t         ,patients_gender\n\t         ,patients_email\n\t         ,patients_phone\n\t         ,patients_birthdate\n\t         ,patients_age\n\t         ,patients_height\n\t         ,patients_weight\n\t         ,patients_address\n\t         ,patients_created_at\n\t         ,CURRENT_TIMESTAMP\n\t         ,patients_info\nFROM PATIENTS\nWHERE patients_id = %s;\nDELETE FROM PATIENTS\nWHERE patients_id = %s;", "regular expression (\"\")"="%s" ("regular expression (\"\")"), "replace string (\"\")"=w107, "replace all? (F)"=TRUE) -> ("result string"=w109:string)  [unwired: 1 in, 1 out]
    }
    frame "restore" {
      n26 = call <vilib>:"Search and Replace Pattern.vi"("string"="INSERT INTO  PATIENTS\n(\n  patients_id\n ,patients_nm\n ,patients_gender\n ,patients_email\n ,patients_phone\n ,patients_birthdate\n ,patients_age\n ,patients_height\n ,patients_weight\n ,patients_address\n ,patients_created_at\n ,patients_updated_at\n ,patients_info\n)\nSELECT patients_id\n\t         ,patients_nm\n\t         ,patients_gender\n\t         ,patients_email\n\t         ,patients_phone\n\t         ,patients_birthdate\n\t         ,patients_age\n\t         ,patients_height\n\t         ,patients_weight\n\t         ,patients_address\n\t         ,patients_created_at\n\t         ,CURRENT_TIMESTAMP\n\t         ,patients_info\nFROM PATIENTS_TRASH\nWHERE patients_id = %s;\nDELETE FROM PATIENTS_TRASH\nWHERE patients_id = %s;", "regular expression (\"\")"="%s" ("regular expression (\"\")"), "replace string (\"\")"=w115, "replace all? (F)"=TRUE) -> ("result string"=w114:string)  [unwired: 1 in, 1 out]
    }
    frame "close" {
      # "x"
    }
  }
  n27 = disable-structure shown="비활성화" {
    frame Disabled {
      (unwired) "-- 'PATIENTS'에서 'PATIENTS_TRASH'로 특정 환자의 데이터 이동\nINSERT INTO PATIENTS_TRASH (patients_id, patients_first_name, patients_last_name, patients_gender, patients_email, patients_phone, patients_birthdate, patients_age, patients_height, patients_weight, patients_address, patients_created_at, patients_updated_at, patients_info)\nSELECT patients_id, patients_first_name, patients_last_name, patients_gender, patients_email, patients_phone, patients_birthdate, patients_age, patients_height, patients_weight, patients_address, patients_created_at, patients_updated_at, patients_info\nFROM PATIENTS\nWHERE patients_id = '%s';\n\n-- 'PATIENTS'에서 해당 환자의 데이터 삭제\nDELETE FROM PATIENTS\nWHERE patients_id = '%s';\n"
      (unwired) "SELECT COUNT(*) AS patients_count\nFROM PATIENTS\nWHERE patients_nm LIKE '%' || '%s' || '%'\n   OR patients_nm LIKE '%' || '%s' || '%'" ("Query")
      (unwired) "INSERT INTO ADMIN_USER \n(\n\t login_id\n\t,user_nm\n\t,user_pw\n\t,user_phone\n\t,user_email\n\t,security_question\n\t,security_answer\n\t,role_id\n) \nVALUES\n(\n\t'%s'\n\t,'%s'\n\t,'%s'\n\t,'%s'\n\t,'%s'\n\t,'%s'\n\t,'%s'\n\t,3\n);"
      (unwired) "SELECT AU.user_id\n\t         ,AU.login_id\n\t         ,AU.user_nm\n\t         ,AU.user_email\n          ,R.role_nm\n\t         ,strftime('%Y-%m-%d', AU.created_at) AS created_at\nFROM ADMIN_USER AU\nJOIN ROLE R ON AU.role_id = R.role_id\nWHERE AU.user_nm LIKE '%' || '%s' || '%'\nORDER BY AU.updated_at DESC \nLIMIT 15 OFFSET (%s - 1) * 15" ("Query")
      # "행의 총 개수"
      # "15개 행 읽기"
      n28 = Format Into String(format string="DELETE FROM ADMIN_USER\nWHERE user_id = '%s';" ("Query")) -> (resulting string=w132:string)  [unwired: 3 in, 1 out]
      n29 = call "comDB.vi"("Query"=w132, "State"=T2."delete") -> ()  [unwired: 5 in, 4 out]
      n30 = call "comDB.vi"("Query"="SELECT AU.user_id\n\t         ,AU.login_id\n\t         ,AU.user_nm\n\t         ,AU.user_email\n          ,R.role_nm\n\t         ,strftime('%Y-%m-%d', AU.created_at) AS created_at\nFROM ADMIN_USER AU\nJOIN ROLE R ON AU.role_id = R.role_id\nWHERE AU.user_nm LIKE '%' || '' || '%'\nORDER BY AU.updated_at DESC \nLIMIT 15 OFFSET (1 - 1) * 15", "State"=T2."getReadList") -> ()  [unwired: 5 in, 4 out]
      n31 = call <vilib>:"Search and Replace Pattern.vi"("string"="\nWHERE AU.user_nm LIKE '%' || '%s' || '%'\nORDER BY AU.updated_at DESC \nLIMIT 15 OFFSET (%s - 1) * 15" ("Query"), "regular expression (\"\")"="%s" ("regular expression (\"\")")) -> ("replace string (\"\")"=w128:string, "result string"=w129:string)  [unwired: 2 in, 1 out]
      n32 = call <vilib>:"Search and Replace Pattern.vi"("string"=w129, "regular expression (\"\")"="%s" ("regular expression (\"\")"), "replace string (\"\")"="1" ("regular expression (\"\")")) -> ()  [unwired: 2 in, 2 out]
      n33 = call "comDB.vi"("Query"="SELECT COUNT(*) AS user_count\nFROM ADMIN_USER; ", "State"=T2."getCount") -> ()  [unwired: 5 in, 4 out]
      n34 = Format Into String(format string="SELECT COUNT(*) AS login_valid\nFROM ADMIN_USER\nWHERE login_id = '%s';") -> (resulting string=w123:string)  [unwired: 3 in, 1 out]
      n35 = call "loginDB.vi"("State"=T3."create") -> ("Query"=w122:string)  [unwired: 7 in, 2 out]
      n36 = call "loginDB.vi"("Query"=w123, "State"=T3."read") -> ()  [unwired: 7 in, 2 out]
    }
    frame Enabled {
    }
  }
  n37 = call "comDB.vi"("error in (no error)"="error in (no error)", "Query"=w10, "State"=w11) -> ("error out"=→"error out":errorcluster, "count"=→"count":i64, "result1DArray"=→"result1DArray":string[], "resultList"=→"resultList":string[][])  [unwired: 4 in]
